vi "Motor driver 1 to 1 11.vi"() -> ()   [LabVIEW 2009]
panel:
  in  "Resource Name":refnum<visa-resource-name>="ASRL8::INSTR"
  out "Motor running":bool
  in  "Withdraw piston":T1={"withdrawal rate"=enum."-8E-05 \"/s"}
  out "internal force gauge (v) starting value":ext=-0.014122 format="%.6f"
  in  "OK":bool
  out "Sent string":string
  in  "Mode":i32(listbox)
  in  "Are you sure? copy 2":bool
  in  "Are you sure?":bool
  out "current reset":ext=1.2236 format="%.6f"
  in  "initial reset":ext=0.1 format="%.2f"
  out "local var: load first time flag":bool=TRUE
  out "internal force gauge (v) current value":ext=-0.014122 format="%.6f"
  in  "Constant load":T2={"set pt"=1.0, "Int"=0.1, "Prop"=0.3, "hi reset limit"=5.0, "total limit"=0.0, "lo reset limit"=5.0} {"lo reset limit" format="%.6f"; "total limit" format="%.2f"; "hi reset limit" format="%.6f"; "Prop" format="%.2f"; "Int" format="%.6f"; "set pt" format="%.6f"}
  in  "Constant displacement rate":T3={"displacement rate"=enum."8E-05 \"/s"}
  in  "Load relaxation":cluster{"Does absolutely nothing":u8, bool}
  in  "stop/go":bool
  out "Active string":string="S "
  out "Read String":string
  out "current selected displacement rate":string="8E-06 \"/s"
  # "Note: use of this VI is probably not a great idea until it is made as current as the 10:1 motor driver"
  # "Just push the STOP buttom, dummy"
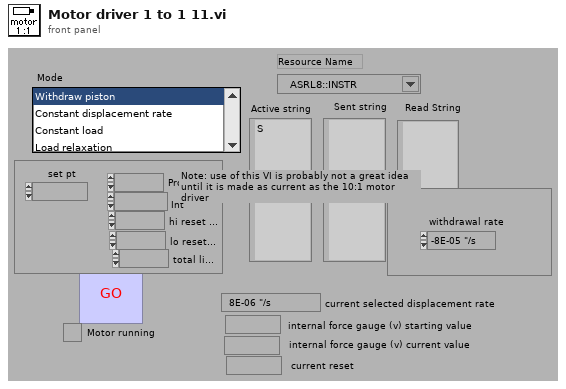
[diagram p1: front panel]
types:
  T1 = cluster{"withdrawal rate":enum16{"-8E-04 \"/s", "-8E-07 \"/s", "-8E-06 \"/s", "-8E-05 \"/s"}}
  T2 = cluster{"set pt":ext, "Int":ext, "Prop":ext, "hi reset limit":ext, "total limit":ext, "lo reset limit":ext}
  T3 = cluster{"displacement rate":enum16{"8E-04 \"/s", "8E-07 \"/s", "8E-06 \"/s", "8E-05 \"/s"}}
  T4 = enum16{"-8E-04 \"/s", "-8E-07 \"/s", "-8E-06 \"/s", "-8E-05 \"/s"}
  T5 = enum16{"8E-04 \"/s", "8E-07 \"/s", "8E-06 \"/s", "8E-05 \"/s"}
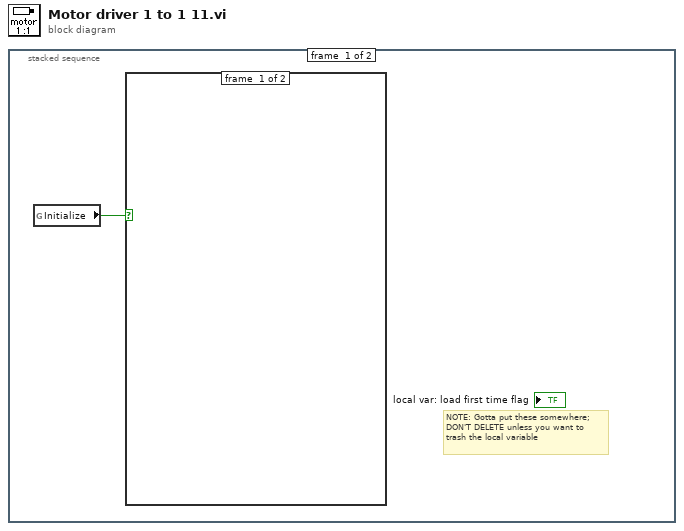
[diagram p0: block diagram]
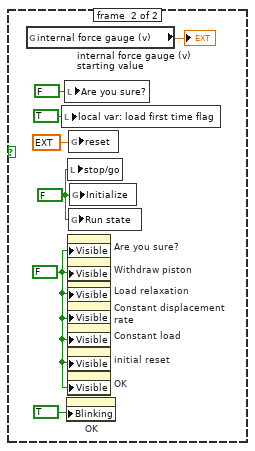
[diagram p2: hidden frame]
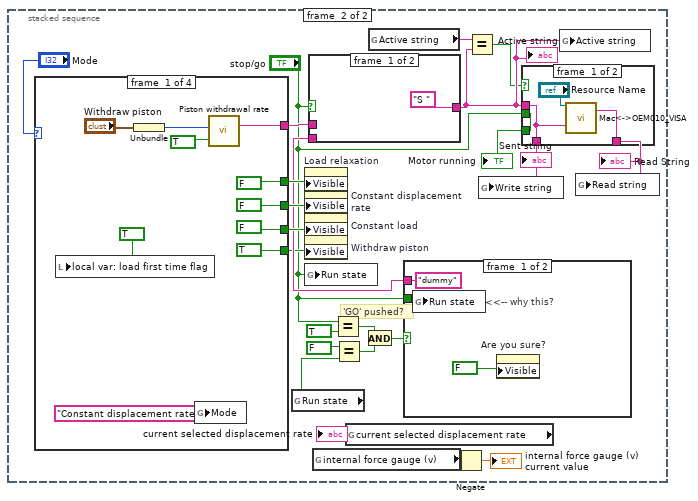
[diagram p3: hidden frame]
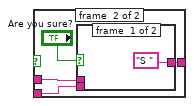
[diagram p4: hidden frame]
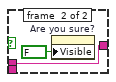
[diagram p5: hidden frame]
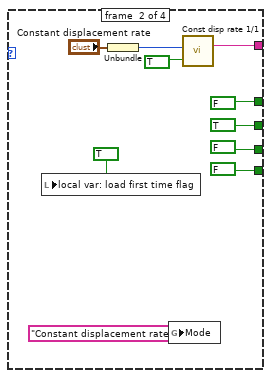
[diagram p6: hidden frame]
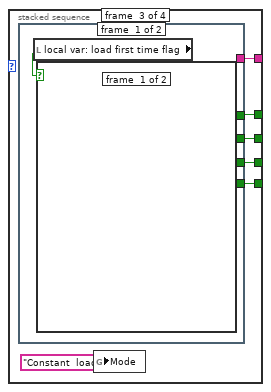
[diagram p7: hidden frame]
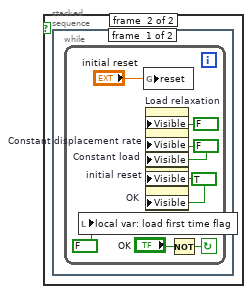
[diagram p8: hidden frame]
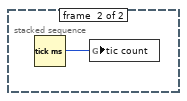
[diagram p9: hidden frame]
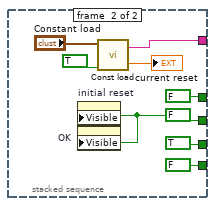
[diagram p10: hidden frame]
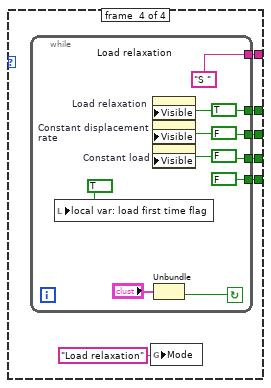
[diagram p11: hidden frame]
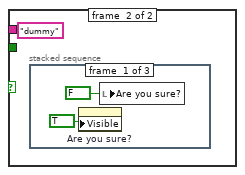
[diagram p12: hidden frame]
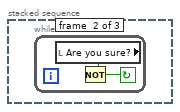
[diagram p13: hidden frame]
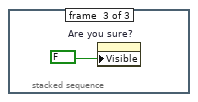
[diagram p14: hidden frame]
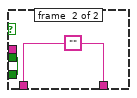
[diagram p15: hidden frame]
diagram:
  n1 = stacked-sequence {
    frame #0 {
      # "NOTE: Gotta put these somewhere; DON'T DELETE unless you want to trash the local variable"
      n2 = global read "Motor drive globals" "Initialize"() -> (w1:bool)
      n3 = case shown="True" w1 {
        frame #0 {
        }
        frame #1 {
          w4 = FALSE
          w2 = FALSE
          n4 = global read "Motor drive globals" "internal force gauge (v)"() -> (→"internal force gauge (v) starting value":ext)
          n5 = local write "local var: load first time flag"(TRUE) -> ()
          n6 = local write "Are you sure?"(FALSE) -> ()
          n7 = property on="OK" class="Boolean"("Blinking"=TRUE) -> ()  [unwired: 2 in, 2 out]
          n8 = local write "stop/go"(w4) -> ()
          n9 = property on="Are you sure?" class="Boolean (strict)"("Visible"=w2) -> ()  [unwired: 2 in, 2 out]
          n10 = property on="Withdraw piston" class="Cluster (strict)"("Visible"=w2) -> ()  [unwired: 2 in, 2 out]
          n11 = property on="Load relaxation" class="Cluster"("Visible"=w2) -> ()  [unwired: 2 in, 2 out]
          n12 = property on="Constant displacement rate" class="Cluster (strict)"("Visible"=w2) -> ()  [unwired: 2 in, 2 out]
          n13 = property on="Constant load" class="Clust (strict)"("Visible"=w2) -> ()  [unwired: 2 in, 2 out]
          n14 = property on="initial reset" class="Digital (strict)"("Visible"=w2) -> ()  [unwired: 2 in, 2 out]
          n15 = property on="OK" class="Boolean"("Visible"=w2) -> ()  [unwired: 2 in, 2 out]
          n16 = global write "Motor drive globals" "reset"(ext 0.0) -> ()
          n17 = global write "Motor drive globals" "Run state"(w4) -> ()
          n18 = global write "Motor drive globals" "Initialize"(w4) -> ()
        }
      }
    }
    frame #1 {
      # "'GO' pushed?"
      n19 = case shown="2" "Mode" {
        tunnel: [w45 w54 w62 w85] -> w24
        tunnel: [FALSE FALSE w65 w88] -> w25
        tunnel: [FALSE TRUE w64 w87] -> w26
        tunnel: [FALSE FALSE w63 w86] -> w27
        tunnel: [TRUE FALSE w60 w83] -> w12
        frame #0 {
          n20 = local write "local var: load first time flag"(TRUE) -> ()
          n21 = Unbundle("Withdraw piston") -> ("withdrawal rate"=w49:T4)
          n22 = global write "Motor drive globals" "Mode"("Constant displacement rate") -> ()
          n23 = call "Piston withdrawal rate"("Start"=TRUE, "withdrawal rate"=w49) -> ("Write String"=w45:string)  [unwired: 1 in]
        }
        frame #1 {
          n24 = local write "local var: load first time flag"(TRUE) -> ()
          n25 = Unbundle("Constant displacement rate") -> ("displacement rate"=w58:T5)
          n26 = global write "Motor drive globals" "Mode"("Constant displacement rate") -> ()
          n27 = call "Const disp rate 1/1"("Start"=TRUE, "displacement rate"=w58) -> ("Write String"=w54:string)  [unwired: 1 in]
        }
        frame #2 {
          n28 = stacked-sequence {
            tunnel: [_ FALSE] -> w65
            tunnel: [_ w76] -> w64
            tunnel: [_ TRUE] -> w63
            tunnel: [_ w77] -> w62
            tunnel: [_ FALSE] -> w60
            frame #0 {
              n29 = local read "local var: load first time flag"() -> (w66:bool)
              n30 = case shown="True" w66 {
                frame #0 {
                }
                frame #1 {
                  n31 = stacked-sequence {
                    frame #0 {
                      n32 = while {
                        stop <- w68 continue-if-true
                        w73 = FALSE
                        w67 = TRUE
                        n33 = local write "local var: load first time flag"(FALSE) -> ()
                        n34 = global write "Motor drive globals" "reset"("initial reset") -> ()
                        n35 = property on="Load relaxation" class="Cluster"("Visible"=FALSE) -> ()  [unwired: 2 in, 2 out]
                        n36 = property on="Constant displacement rate" class="Cluster (strict)"("Visible"=w73) -> ()  [unwired: 2 in, 2 out]
                        n37 = property on="Constant load" class="Clust (strict)"("Visible"=w73) -> ()  [unwired: 2 in, 2 out]
                        n38 = property on="initial reset" class="Digital (strict)"("Visible"=w67) -> ()  [unwired: 2 in, 2 out]
                        n39 = property on="OK" class="Boolean"("Visible"=w67) -> ()  [unwired: 2 in, 2 out]
                        n40 = Not(x="OK") -> (.not. x?=w68:bool)
                      }
                    }
                    frame #1 {
                      n41 = Tick Count (ms)() -> (millisecond timer value=w74:u32)
                      n42 = global write "Motor drive globals" "tic count"(w74) -> ()
                    }
                  }
                }
              }
            }
            frame #1 {
              w76 = FALSE
              n43 = property on="initial reset" class="Digital (strict)"("Visible"=w76) -> ()  [unwired: 2 in, 2 out]
              n44 = property on="OK" class="Boolean"("Visible"=w76) -> ()  [unwired: 2 in, 2 out]
              n45 = call "Const load"("send values"=TRUE, 5:"Constant load") -> ("current reset"=→"current reset":ext, "Write String"=w77:string)  [unwired: 2 in]
            }
          }
          n46 = global write "Motor drive globals" "Mode"("Constant  load") -> ()
        }
        frame #3 {
          n47 = while {
            tunnel: [w95] -> w88
            tunnel: [w94] -> w87
            tunnel: [w93] -> w86
            tunnel: ["S "] -> w85
            tunnel: [FALSE] -> w83
            stop <- w90 continue-if-true
            w95 = TRUE
            w94 = FALSE
            w93 = FALSE
            n48 = local write "local var: load first time flag"(TRUE) -> ()
            n49 = property on="Load relaxation" class="Cluster"("Visible"=w95) -> ()  [unwired: 2 in, 2 out]
            n50 = property on="Constant displacement rate" class="Cluster (strict)"("Visible"=w94) -> ()  [unwired: 2 in, 2 out]
            n51 = property on="Constant load" class="Clust (strict)"("Visible"=w93) -> ()  [unwired: 2 in, 2 out]
            n52 = Unbundle("Load relaxation") -> (w90:bool)  [unwired: 1 out]
          }
          n53 = global write "Motor drive globals" "Mode"("Load relaxation") -> ()
        }
      }
      n54 = global read "Motor drive globals" "Run state"() -> (w11:bool)
      n55 = property on="Load relaxation" class="Cluster"("Visible"=w25) -> ()  [unwired: 2 in, 2 out]
      n56 = property on="Constant displacement rate" class="Cluster (strict)"("Visible"=w26) -> ()  [unwired: 2 in, 2 out]
      n57 = property on="Constant load" class="Clust (strict)"("Visible"=w27) -> ()  [unwired: 2 in, 2 out]
      n58 = property on="Withdraw piston" class="Cluster (strict)"("Visible"=w12) -> ()  [unwired: 2 in, 2 out]
      n59 = global write "Motor drive globals" "Run state"("stop/go") -> ()
      n60 = global read "Motor drive globals" "internal force gauge (v)"() -> (w19:ext)
      n61 = Equal?(x="stop/go", y=TRUE) -> (x = y?=w15:bool)
      n62 = Equal?(x=FALSE, y=w11) -> (x = y?=w14:bool)
      n63 = global read "Motor drive globals" "current selected displacement rate"() -> (→"current selected displacement rate":string)
      n64 = And(x=w15, y=w14) -> (x .and. y?=w18:bool)
      n65 = global read "Motor drive globals" "Active string"() -> (w31:string)
      n66 = case shown="False" w18 {
        tunnel: ["dummy" "dummy"] -> w13
        tunnel: "stop/go" -> [w97 _]
        frame #0 {
          # "<<-- why this?"
          n67 = global write "Motor drive globals" "Run state"(w97) -> ()
          n68 = property on="Are you sure?" class="Boolean (strict)"("Visible"=FALSE) -> ()  [unwired: 2 in, 2 out]
        }
        frame #1 {
          n69 = stacked-sequence {
            frame #0 {
              n70 = property on="Are you sure?" class="Boolean (strict)"("Visible"=TRUE) -> ()  [unwired: 2 in, 2 out]
              n71 = local write "Are you sure?"(FALSE) -> ()
            }
            frame #1 {
              n72 = while {
                stop <- w103 continue-if-true
                n73 = local read "Are you sure?"() -> (w104:bool)
                n74 = Not(x=w104) -> (.not. x?=w103:bool)
              }
            }
            frame #2 {
              n75 = property on="Are you sure?" class="Boolean (strict)"("Visible"=FALSE) -> ()  [unwired: 2 in, 2 out]
              n76 = property on="Are you sure? copy 2" class="Boolean (strict)"("Visible"=FALSE) -> ()  [unwired: 2 in, 2 out]
            }
          }
        }
      }
      n77 = case shown="True" "stop/go" {
        tunnel: w24 -> [_ w35]
        tunnel: w13 -> [_ w33]
        tunnel: ["S " w34] -> w30
        frame #0 {
        }
        frame #1 {
          n78 = case shown="False" "Are you sure?" {
            tunnel: w35 -> [_ w38]
            tunnel: ["S " w38] -> w34
            tunnel: w33 -> [_ _]
            frame #0 {
            }
            frame #1 {
              n79 = property on="Are you sure?" class="Boolean (strict)"("Visible"=FALSE) -> ()  [unwired: 2 in, 2 out]
            }
          }
        }
      }
      "Active string" <- w30
      n80 = Negate(x=w19) -> (-x=→"internal force gauge (v) current value":ext)
      n81 = Equal?(x=w31, y=w30) -> (x = y?=w29:bool)
      n82 = case shown="False" w29 {
        tunnel: w30 -> [w107 _]
        tunnel: [w109 w112] -> w22
        tunnel: [w107 w112] -> w21
        tunnel: [w110 w111] -> w10
        tunnel: "stop/go" -> [w110 w111]
        frame #0 {
          n83 = call "Mac<->OEM010_VISA"("Resource Name"="Resource Name", "Serial Write"=w107) -> ("Serial Read"=w109:string)  [unwired: 12 in, 5 out]
        }
        frame #1 {
          w112 = ""
        }
      }
      "Read String" <- w22
      "Sent string" <- w21
      "Motor running" <- w10
      n84 = global write "Motor drive globals" "Write string"(w21) -> ()
      n85 = global write "Motor drive globals" "Active string"(w30) -> ()
      n86 = global write "Motor drive globals" "Read string"(w22) -> ()
    }
  }
